vi "Refresh Control.vi"(8 "error in (no error)":errorcluster, 11 "Analog-Output in":refnum<class "Analog-Output.lvclass">) -> (0 "error out":errorcluster, 3 "Analog-Output out":refnum<class "Analog-Output.lvclass">)   [LabVIEW 2019, in "Analog-Output.lvlib" / "Analog-Output.lvclass"]
uses:
  Library/Analog-Output.lvclass
  Library/Analog-Output.lvclass/Analog-Output.ctl
  Accessors/Read Settings.vi
  Accessors/Read Settings_All.vi
  Accessors/Read Measured Table.vi
  Accessors/Write Settings.vi
  Accessors/Write Measured Table.vi
  Accessors/Read All Voltages.vi
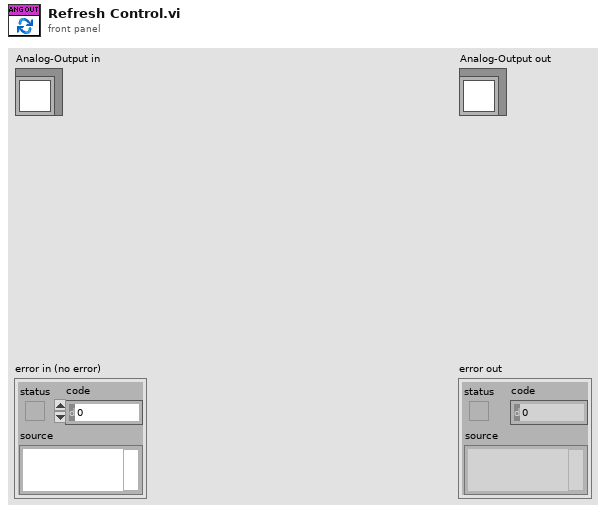
[diagram p1: front panel]
types:
  T1 = typedef "Analog-Output.lvlib/Analog-Output.lvclass/Settings.ctl" = cluster{"Voltage":dbl}
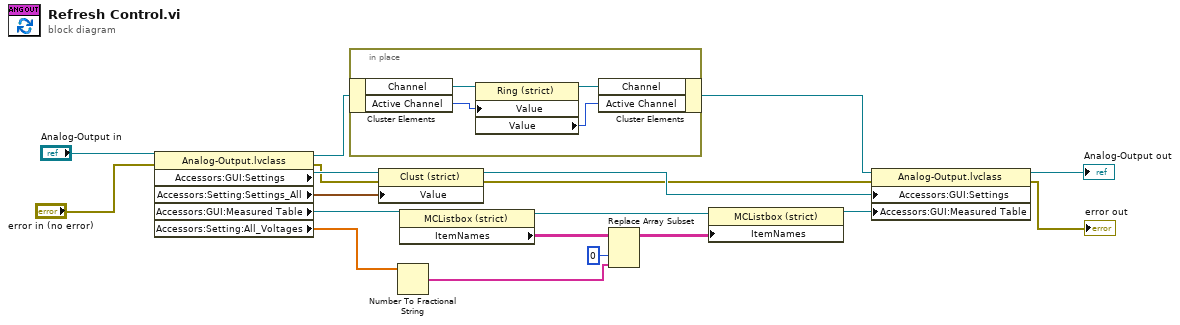
[diagram p0: block diagram]
diagram:
  n1 = property class="Analog-Output.lvclass"(reference="Analog-Output in", error in="error in (no error)") -> (reference out=w16:refnum<class "Analog-Output.lvclass">, error out=w11:errorcluster, "Accessors:GUI:Settings"=w18:refnum<vi>, "Accessors:Setting:Settings_All"=w17:T1, "Accessors:GUI:Measured Table"=w7:refnum<vi>, "Accessors:Setting:All_Voltages"=w2:dbl[])
  n2 = in-place {
    n3 = in-place-cluster #1(w16) -> ("Channel"=w23:refnum<vi>, "Active Channel"=w21:u32)
    n4 = property class="Ring (strict)"(reference=w23, "Value"=w21) -> (reference out=w22:refnum<vi>, "Value"=w20:u16)  [unwired: 1 in, 1 out]
    n5 = in-place-cluster #1("Channel"=w22, "Active Channel"=w20) -> (w15:refnum<class "Analog-Output.lvclass">)
  }
  n6 = property class="Clust (strict)"(reference=w18, error in=w11, "Value"=w17) -> (reference out=w13:refnum<vi>, error out=w10:errorcluster)
  n7 = Number To Fractional String(number=w2) -> (F-format string=w1:string[])  [unwired: 3 in]
  n8 = property class="MCListbox (strict)"(reference=w7) -> (reference out=w6:refnum<vi>, "ItemNames"=w5:string[][])  [unwired: 1 in, 1 out]
  n9 = Replace Array Subset(array=w5, new element=w1, index (col)=0 ("disabled index (col)")) -> (w4:string[][])  [unwired: 1 in]
  n10 = property class="MCListbox (strict)"(reference=w6, "ItemNames"=w4) -> (reference out=w8:refnum<vi>)  [unwired: 1 in, 1 out]
  n11 = property class="Analog-Output.lvclass"(reference=w15, error in=w10, "Accessors:GUI:Settings"=w13, "Accessors:GUI:Measured Table"=w8) -> (reference out=→"Analog-Output out":refnum<class "Analog-Output.lvclass">, error out=→"error out":errorcluster)
